vi "data out of range.vi"(8 "error in":errorcluster, 9 "source":string="slave not available.vi", 10 "byte":i32, 11 "slave":i8) -> (0 "error out":errorcluster)   [LabVIEW 2013, in "Profibus Module runtime.lvclass"]
uses:
  Profibus Module runtime.lvclass
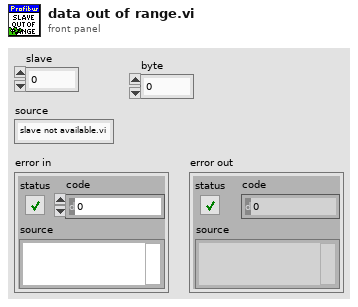
[diagram p1: front panel]
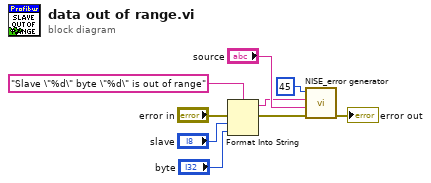
[diagram p0: block diagram]
diagram:
  n1 = Format Into String(format string="Slave \"%d\" byte \"%d\" is out of range", error in="error in", "slave", "byte") -> (resulting string=w3:string, error out=w5:errorcluster)  [unwired: 1 in]
  n2 = call <vilib>:"NISE_error generator.vi"("error in"=w5, "source"="source", "append error message"=w3, "error code (0)"=45) -> ("error out"=→"error out":errorcluster)  [unwired: 5 in]
